vi "NewBoardc.vi"() -> ()   [LabVIEW 2014]
uses:
  <vilib>/Instr/_visa.llb/VISA Configure Serial Port (Instr).vi
panel:
  out "Array 3":string[](array[string])
  out "Array 2":T1(array[cluster]) {"Current Raw" format="%x"; "Detector Raw" format="%x"}
  in  "stop":bool
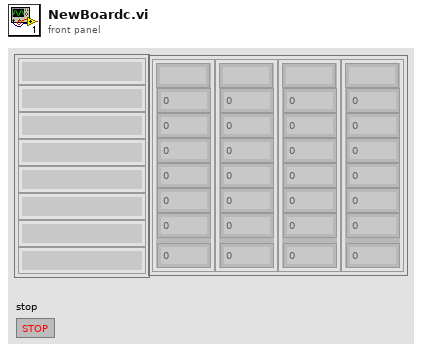
[diagram p1: front panel]
types:
  T1 = cluster{"Channel":string, "Detector Raw":u16, "Detector Adjusted":dbl, "Current Raw":u16, "Current Adjusted":dbl, "Temperature":dbl, "Humidity":dbl, "Calculated\nCO2":dbl}[]
  T2 = cluster{"Channel":string, "Detector Raw":u16, "Detector Adjusted":dbl, "Current Raw":u16, "Current Adjusted":dbl, "Temperature":dbl, "Humidity":dbl, "Calculated\nCO2":dbl}
  T3 = cluster{"Detector":cluster{"String":string, "Raw":u16, "Adjusted":dbl}, "Current":cluster{"String":string, "Raw":u16, "Adjusted":dbl}, "Sensor\nTemperature":dbl, "Sensor\nHumidity":dbl, "Calculated\nCO2":dbl}
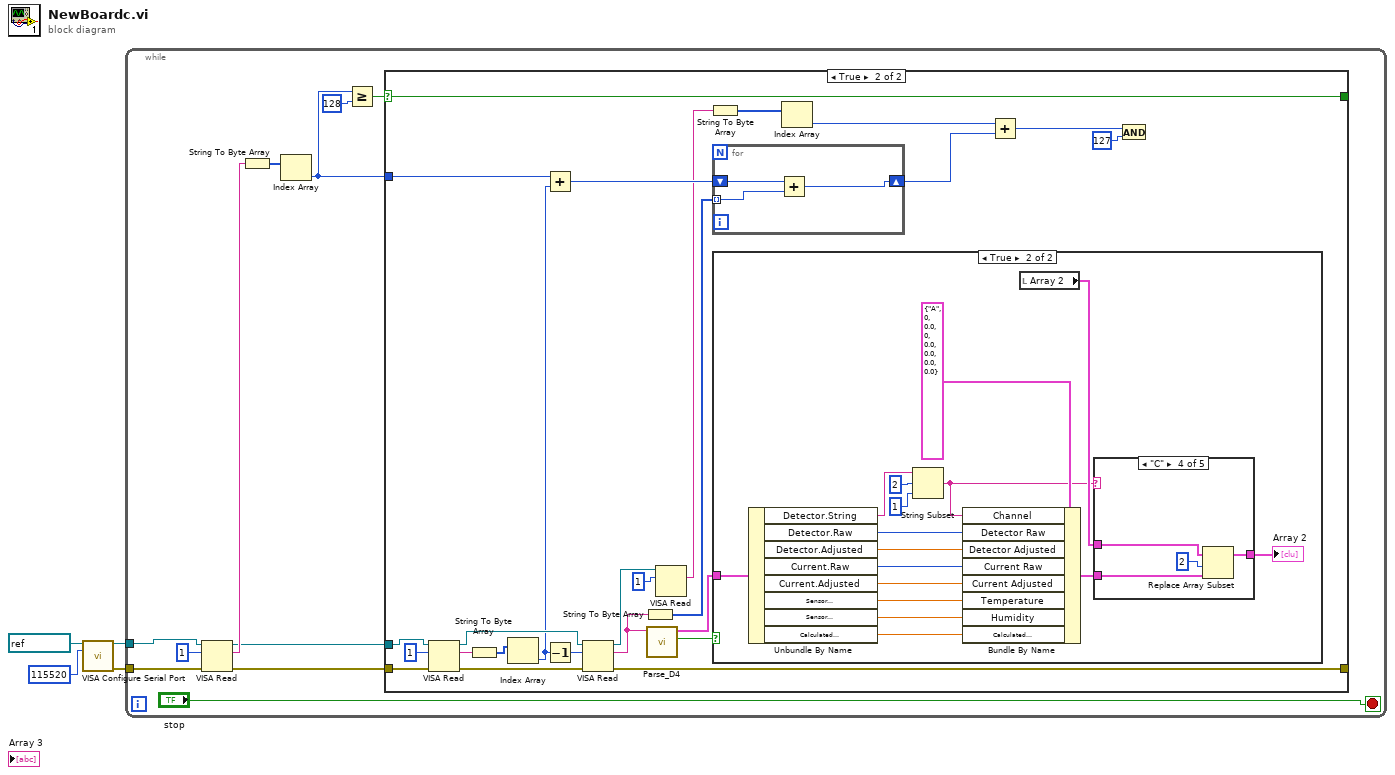
[diagram p0: block diagram]
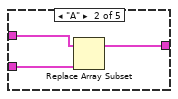
[diagram p5: hidden frame]
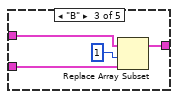
[diagram p6: hidden frame]
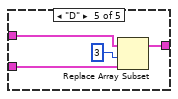
[diagram p7: hidden frame]
diagram:
  n1 = call-poly "VISA Configure Serial Port"("VISA resource name"=refnum<visa-resource-name> "COM7" ("Serial Port.VISA resource name"), "baud rate (9600)"=u32 115520 ("Serial Port.baud rate")) -> ("VISA resource name out"=w2:refnum<visa-resource-name>, "error out"=w1:errorcluster)  [unwired: 12 in]
  n2 = while {
    tunnel: w2 -> [w15]
    tunnel: w1 -> [w12]
    stop <- "stop" stop-if-true
    n3 = VISA Read(VISA resource name=w15, byte count=u32 1, error in (no error)=w12) -> (VISA resource name out=w7:refnum<visa-resource-name>, read buffer=w11:string, error out=w6:errorcluster)  [unwired: 1 out]
    n4 = String To Byte Array(string=w11) -> (unsigned byte array=w10:u8[])
    n5 = Index Array(array=w10) -> (element=w5:u8)  [unwired: 1 in]
    n6 = Greater Or Equal?(x=w5, y=u8 128) -> (x >= y?=w8:bool)
    n7 = case shown="True" w8 {
      selector: w8 -> [_ w36]
      tunnel: w7 -> [_ w41]
      tunnel: w6 -> [w16 w39]
      tunnel: [w16 w33] -> _
      tunnel: [_ w36] -> _
      tunnel: w5 -> [_ w29]
      frame False {
      }
      frame True {
        n8 = VISA Read(VISA resource name=w41, byte count=u32 1, error in (no error)=w39) -> (VISA resource name out=w35:refnum<visa-resource-name>, read buffer=w38:string, error out=w34:errorcluster)  [unwired: 1 out]
        n9 = String To Byte Array(string=w38) -> (unsigned byte array=w37:u8[])
        n10 = Index Array(array=w37) -> (element=w28:u8)  [unwired: 1 in]
        n11 = Add(x=w29, y=w28) -> (x+y=w26:u8)
        n12 = Decrement(x=w28) -> (x-1=w32:u8)
        n13 = VISA Read(VISA resource name=w35, byte count=w32, error in (no error)=w34) -> (VISA resource name out=w31:refnum<visa-resource-name>, read buffer=w19:string, error out=w33:errorcluster)  [unwired: 1 out]
        n14 = String To Byte Array(string=w19) -> (unsigned byte array=w27:u8[])
        n15 = call "Parse_D4.vi"("read buffer"=w19) -> ("D4"=w17:bool, "Data"=w18:T3)  [unwired: 9 in]
        n16 = VISA Read(VISA resource name=w31, byte count=u32 1) -> (read buffer=w25:string)  [unwired: 1 in, 3 out]
        n17 = String To Byte Array(string=w25) -> (unsigned byte array=w24:u8[])
        n18 = for {
          tunnel: w27 -> [w75] mode=indexing
          shift-right: [w74] -> w21
          shift-left: w26 -> [w76]
          n19 = Add(x=w76, y=w75) -> (x+y=w74:u8)
        }
        n20 = case shown="True" w17 {
          tunnel: w18 -> [_ w57]
          frame False {
          }
          frame True {
            n21 = Unbundle By Name(w57) -> ("Detector.String"=w43:string, "Detector.Raw"=w55:u16, "Detector.Adjusted"=w54:dbl, "Current.Raw"=w53:u16, "Current.Adjusted"=w52:dbl, "Sensor\nTemperature"=w51:dbl, "Sensor\nHumidity"=w50:dbl, "Calculated\nCO2"=w49:dbl)
            n22 = String Subset(string=w43, offset (0)=2, length (rest)=1 ("length (rest)")) -> (substring=w42:string)
            n23 = Bundle By Name(cluster=T2 {"Channel"="A", "Detector Raw"=0, "Detector Adjusted"=0.0, "Current Raw"=0, "Current Adjusted"=0.0, "Temperature"=0.0, "Humidity"=0.0, "Calculated\nCO2"=0.0} ("Cluster"), "Channel"=w42, "Detector Raw"=w55, "Detector Adjusted"=w54, "Current Raw"=w53, "Current Adjusted"=w52, "Temperature"=w51, "Humidity"=w50, "Calculated\nCO2"=w49) -> (w48:T2)
            n24 = local read "Array 2"() -> (w45:T1)
            n25 = case shown="\"C\"" w42 {
              tunnel: w48 -> [_ w61 w64 w68 w72]
              tunnel: w45 -> [w58 w60 w65 w69 w73]
              tunnel: [w58 w59 w62 w66 w70] -> w44
              frame "False", Default {
              }
              frame "A" {
                n26 = Replace Array Subset(array=w60, new element=w61) -> (w59:T1)  [unwired: 1 in]
              }
              frame "B" {
                n27 = Replace Array Subset(array=w65, new element=w64, index=1) -> (w62:T1)
              }
              frame "C" {
                n28 = Replace Array Subset(array=w69, new element=w68, index=2) -> (w66:T1)
              }
              frame "D" {
                n29 = Replace Array Subset(array=w73, new element=w72, index=3) -> (w70:T1)
              }
            }
            "Array 2" <- w44
          }
        }
        n30 = Index Array(array=w24) -> (element=w22:u8)  [unwired: 1 in]
        n31 = Add(x=w22, y=w21) -> (x+y=w20:u8)
        n32 = And(x=w20, y=u8 127) -> ()  [unwired: 1 out]
      }
    }
  }
